vi "RSZVB Set Fast Multiport Correction.vi"(8 "error in (no error)":errorcluster {"code" format="%.0x"}, 10 "Fast Multiport Correction (On   (1)":bool, 11 "VISA session":refnum<visa-resource-name>) -> (0 "error out":errorcluster {"code" format="%.0x"}, 3 "dup VISA session":refnum<visa-resource-name>)   [LabVIEW 2011]
doc: "This VI enables or disables Fast Multiport Correction.\n\nRemote-control command(s):\nSYSTem:CORRection:FMPort[:STATe]"
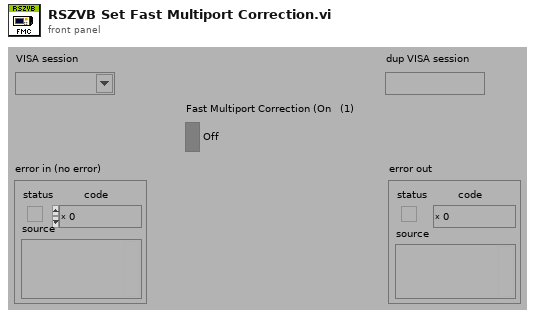
[diagram p1: front panel]
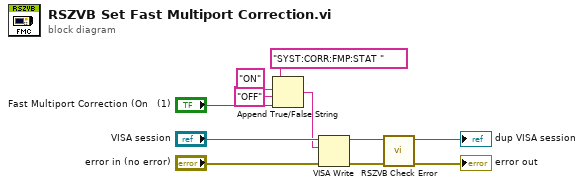
[diagram p0: block diagram]
diagram:
  n1 = Append True/False String(1:"Fast Multiport Correction (On   (1)", 2:"OFF" ("false string"), 3:"ON" ("true string"), 4:"SYST:CORR:FMP:STAT " ("string (\"\")")) -> (0:w5:string)
  n2 = VISA Write(VISA resource name="VISA session", write buffer=w5, error in (no error)="error in (no error)") -> (VISA resource name out=w3:refnum<visa-resource-name>, error out=w4:errorcluster)  [unwired: 1 out]
  n3 = call "RSZVB Check Error.vi"("error in (no error)"=w4, "VISA session"=w3) -> ("error out"=→"error out":errorcluster, "dup VISA session"=→"dup VISA session":refnum<visa-resource-name>)  [unwired: 8 in]
